vi "test.vi"() -> ()   [LabVIEW 2017]
panel:
  out "number":u64
  in  "Boolean array 2":bool[](array[boolean])
  out "Boolean array":bool[](array[boolean])
  in  "Array 2":bool[](array[boolean])
  in  "Array":bool[](array[boolean])
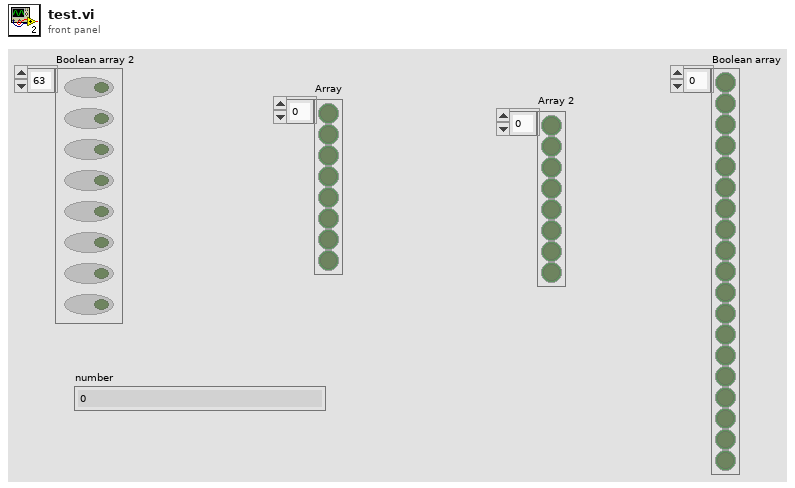
[diagram p1: front panel]
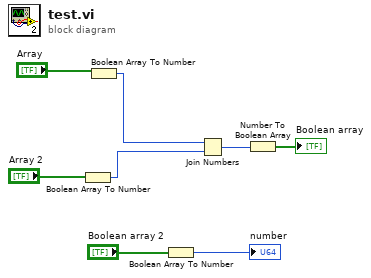
[diagram p0: block diagram]
diagram:
  n1 = Boolean Array To Number(Boolean array="Array 2") -> (number=w5:u8)
  n2 = Boolean Array To Number(Boolean array="Array") -> (number=w6:u8)
  n3 = Boolean Array To Number(Boolean array="Boolean array 2") -> (number=→"number":u64)
  n4 = Join Numbers(hi=w6, lo=w5) -> ((hi.lo)=w4:u16)
  n5 = Number To Boolean Array(number=w4) -> (Boolean array=→"Boolean array":bool[])
